vi "Create Report.vi"(5 "Test Info":T1, 7 "Test Results":T9, 8 "error in (no error)":errorcluster, 9 "Filepath":path, 10 "Test Config":T2, 11 "Report In":refnum<class "Report.lvclass">) -> (0 "error out":errorcluster, 3 "Report Out":refnum<class "Report.lvclass">)   [LabVIEW 2015, in "Report.lvclass"]
uses:
  Report.lvclass
  Tests/Controls/Step Result.ctl
  Tests/Controls/Test Results.ctl
  Tests/Controls/Test Timing.ctl
  Tests/Controls/Vaccum Thresholds.ctl
  Tests/Controls/Vacuum Test.ctl
  Tests/Controls/Helium Thresholds.ctl
  Tests/Controls/Helium Test.ctl
  Tests/Controls/Test Information.ctl
  Tests/Controls/Startup Thresholds.ctl
  Tests/Controls/Startup Test.ctl
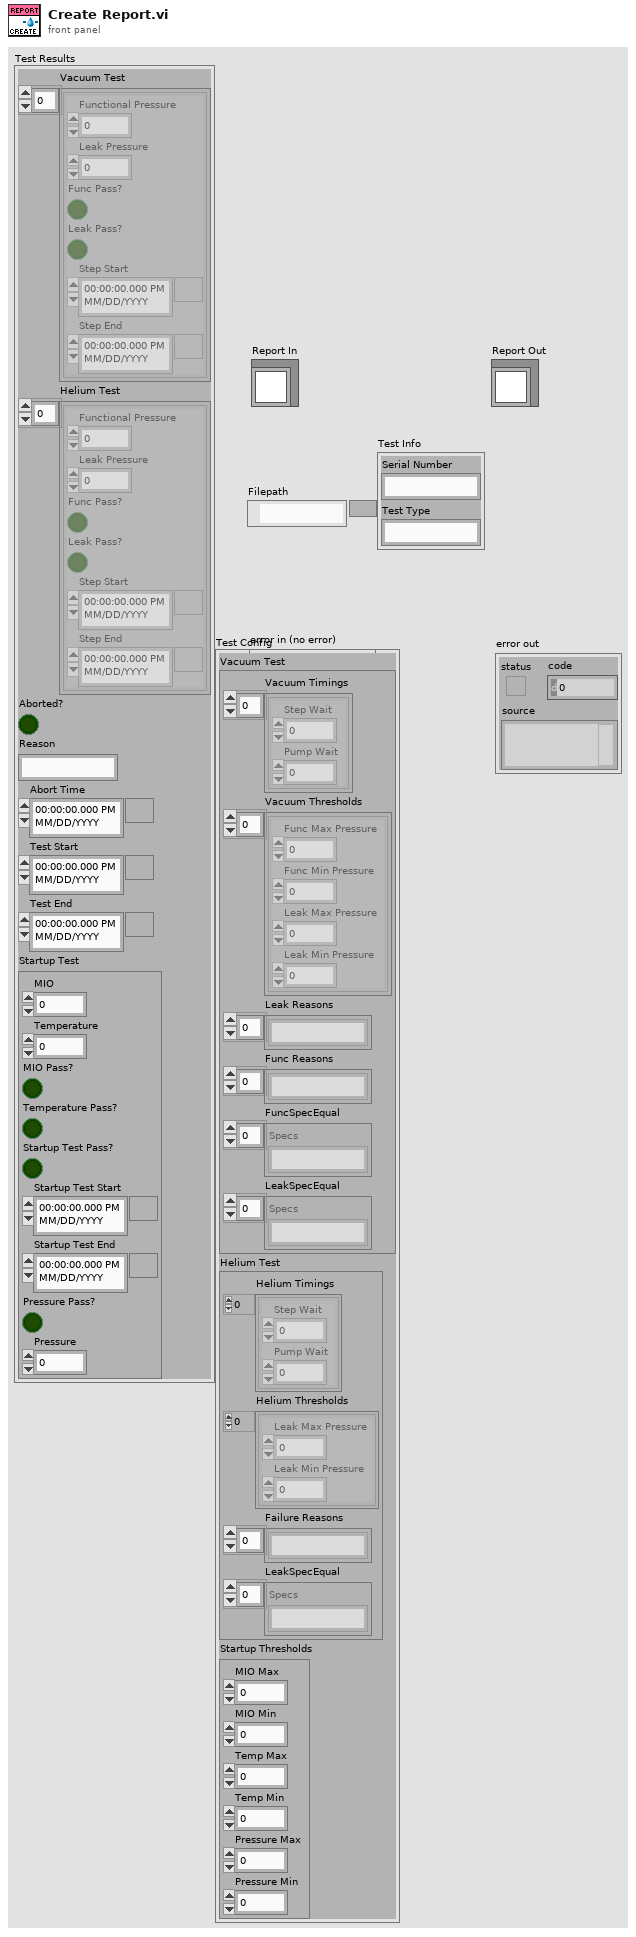
[diagram p1: front panel]
types:
  T1 = cluster{"Serial Number":string, "Test Type":string}
  T2 = typedef "Test Information.ctl" = cluster{"Vacuum Test":T3, "Helium Test":T6, "Startup Thresholds":T8}
  T3 = typedef "Vacuum Test.ctl" = cluster{"Vacuum Timings":T4[], "Vacuum Thresholds":T5[], "Leak Reasons":string[], "Func Reasons":string[], "FuncSpecEqual":string[], "LeakSpecEqual":string[]}
  T4 = typedef "Test Timing.ctl" = cluster{"Step Wait":dbl, "Pump Wait":dbl}
  T5 = typedef "Vaccum Thresholds.ctl" = cluster{"Func Max Pressure":dbl, "Func Min Pressure":dbl, "Leak Max Pressure":dbl, "Leak Min Pressure":dbl}
  T6 = typedef "Helium Test.ctl" = cluster{"Helium Timings":T4[], "Helium Thresholds":T7[], "Failure Reasons":string[], "LeakSpecEqual":string[]}
  T7 = typedef "Helium Thresholds.ctl" = cluster{"Leak Max Pressure":dbl, "Leak Min Pressure":dbl}
  T8 = typedef "Startup Thresholds.ctl" = cluster{"MIO Max":dbl, "MIO Min":dbl, "Temp Max":dbl, "Temp Min":dbl, "Pressure Max":dbl, "Pressure Min":dbl}
  T9 = typedef "Test Results.ctl" = cluster{"Vacuum Test":T10[], "Helium Test":T10[], "Aborted?":bool, "Reason":string, "Abort Time":timestamp, "Test Start":timestamp, "Test End":timestamp, "Startup Test":T11}
  T10 = typedef "Step Result.ctl" = cluster{"Functional Pressure":dbl, "Leak Pressure":dbl, "Func Pass?":bool, "Leak Pass?":bool, "Step Start":timestamp, "Step End":timestamp}
  T11 = typedef "Startup Test.ctl" = cluster{"MIO":dbl, "Temperature":dbl, "MIO Pass?":bool, "Temperature Pass?":bool, "Startup Test Pass?":bool, "Startup Test Start":timestamp, "Startup Test End":timestamp, "Pressure Pass?":bool, "Pressure":dbl}
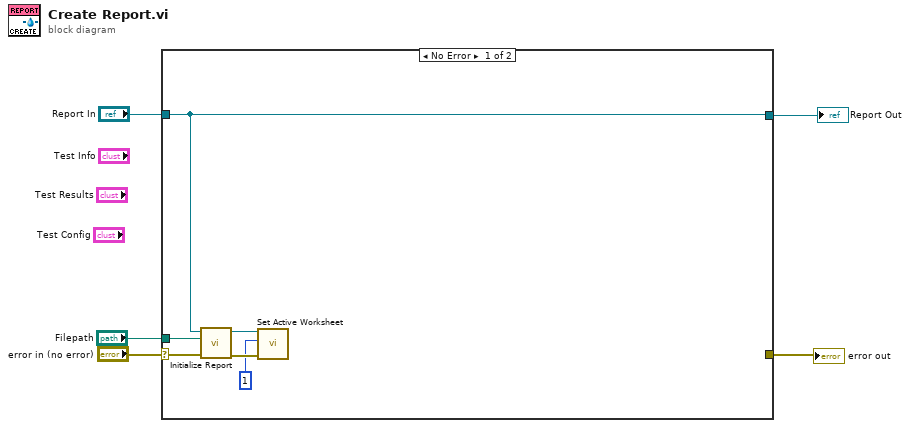
[diagram p0: block diagram]
diagram:
  n1 = case shown="No Error" "error in (no error)" {
    selector: "error in (no error)" -> [w12 w14]
    tunnel: [w6 w14] -> w5
    tunnel: "Report In" -> [w11 w13]
    tunnel: [w11 w13] -> w1
    tunnel: "Filepath" -> [w10 _]
    frame No Error {
      n2 = call "Initialize Report.vi"("error in (no error)"=w12, "Filepath"=w10, "Report In"=w11) -> ("error out"=w8:errorcluster, "Report Out"=w9:refnum<class "Report.lvclass">)  [unwired: 7 in]
      n3 = call "Set Active Worksheet.vi"("error in (no error)"=w8, "Index"=1, "Report In"=w9) -> ()  [unwired: 7 in, 2 out]
    }
    frame Error {
    }
  }
  "error out" <- w5
  "Report Out" <- w1
